vi "Configure Parameter to Measure.vi"(8 "error in (no error)":errorcluster, 10 "Sparameters (string)":string[](array[string]), 11 "VNA-CMT S2 S4 in":refnum<class "VNA-CMT S2 S4.lvclass">) -> (0 "error out":errorcluster, 3 "VNA-CMT S2 S4 out":refnum<class "VNA-CMT S2 S4.lvclass">)   [LabVIEW 2020, in "VNA-CMT S2 S4.lvclass"]
uses:
  VNA-CMT S2 S4.lvclass
  C:/Sandbox/RF Bench/Source Code/WiSpry Test Framework/Instruments/Instrument.lvclass
  Instrument.lvclass/Instrument.ctl
  Instrument.lvclass
  <instrlib>/CMT S2 and S4 VNA/CMT S2 and S4 VNA.lvlib
panel:
  in  "Measurement Parameters (0: S11)":u16(ring) items=["S11", "S21", "S31", "S41", "S12", "S22", "S32", "S42", "S13", "S23", "S33", "S43", "S14", "S24", "S34", "S44", "A", "B", "C", "D", "R1", "R2", "R3", "R4", "T1", "T2", "T3", "T4"]
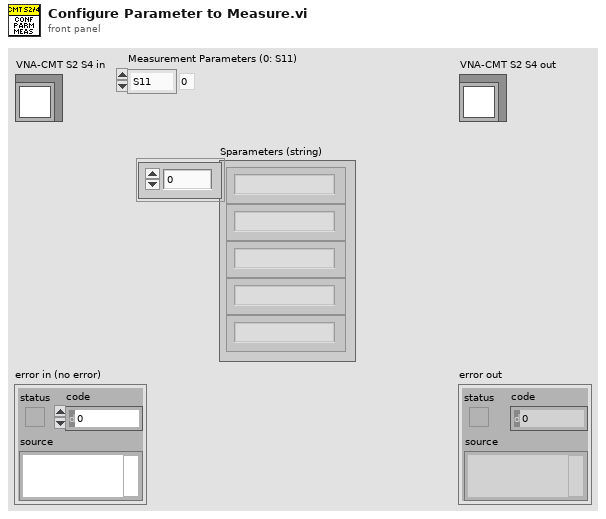
[diagram p1: front panel]
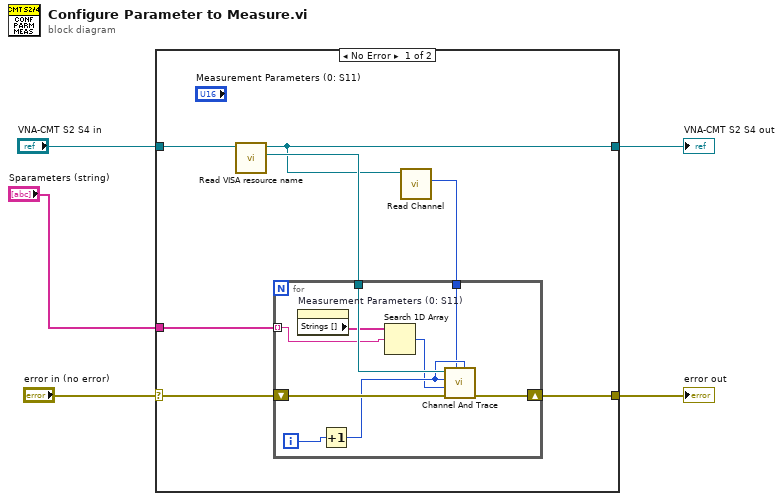
[diagram p0: block diagram]
diagram:
  n1 = case shown="No Error" "error in (no error)" {
    selector: "error in (no error)" -> [w11 w22]
    tunnel: "VNA-CMT S2 S4 in" -> [w12 w23]
    tunnel: [w6 w23] -> w2
    tunnel: [w9 w22] -> w5
    tunnel: "Sparameters (string)" -> [w8 _]
    frame No Error {
      n2 = call "Read VISA resource name.vi"("Instrument in"=w12) -> ("VISA resource name"=w10:refnum<visa-resource-name>, "Instrument out"=w6:refnum<class "VNA-CMT S2 S4.lvclass">)  [unwired: 9 in]
      n3 = call-dynamic "Read Channel.vi"("Vector Network Analyzer in"=w6) -> ("Channel"=w7:i32)  [unwired: 9 in, 1 out]
      n4 = for {
        tunnel: w10 -> [w20]
        shift-right: [w19] -> w9
        shift-left: w11 -> [w21]
        tunnel: w8 -> [w15] mode=indexing
        tunnel: w7 -> [w13]
        i -> [w18]
        n5 = property on="Measurement Parameters (0: S11)" class="Ring (strict)"() -> ("Strings []"=w16:string[])  [unwired: 2 in, 2 out]
        n6 = Increment(x=w18) -> (x+1=w17:i32)
        n7 = Search 1D Array(1D array=w16, element=w15) -> (index of element=w14:i32)  [unwired: 1 in]
        n8 = call <instrlib>:"Channel And Trace.vi"("Active Trace (1)"=w17, "Active Channel (1)"=w13, "error in (no error)"=w21, "Measurement Parameters (0: S11)"=w14, "Number of Traces (1)"=w17, "VISA resource name"=w20) -> ("error out"=w19:errorcluster)  [unwired: 4 in, 1 out]
      }
    }
    frame Error {
    }
  }
  "error out" <- w5
  "VNA-CMT S2 S4 out" <- w2
